vi "OAT Verify Resampled Signal (OMP, Multi Channels).vi"(0 "resampled signal":cluster{"r0":dbl, "dr":dbl, "Y":dbl[]}[](array[cluster]) {"r0" format="%.2p"; "dr" format="%.2p"; "Y" format="%.2f"}, 1 "reset in (T)":bool=TRUE, 5 "X axis selection":u16(ring)=2 items=["Time", "Revolution", "RPM"], 7 "orders to compute (1.0)":dbl[](array[numeric])=[1.0] format="%.2f", 9 "bandwidth [order]":dbl=1.0 format="%.2f", 11 "error in (no error)":errorcluster) -> (3 "reset out (T)":bool=TRUE, 4 "resampled signal out":cluster{"r0":dbl, "dr":dbl, "Y":dbl[]}[](array[cluster]), 6 "X axis selection out":u16(ring)=2 items=["Time", "Revolution", "RPM"], 8 "orders to compute (1.0) out":dbl[](array[numeric])=[1.0] format="%.2f", 10 "bandwidth [order] out":dbl=1.0 format="%.2f", 15 "error out":errorcluster)   [LabVIEW 2017, in "SoundVib_Resampling.lvlib"]
uses:
  <vilib>/addons/Sound and Vibration/Order Analysis/Resample Order Tracking/SoundVib_Resampling.lvlib
  <vilib>/addons/Sound and Vibration/Order Analysis/Resample Order Tracking/SubVIs/OAT Verify Resampled Signal (Multi Channels).vi
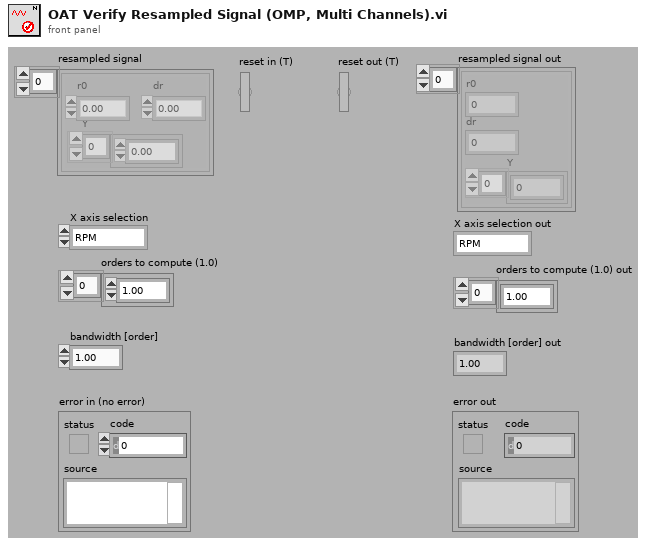
[diagram p1: front panel]
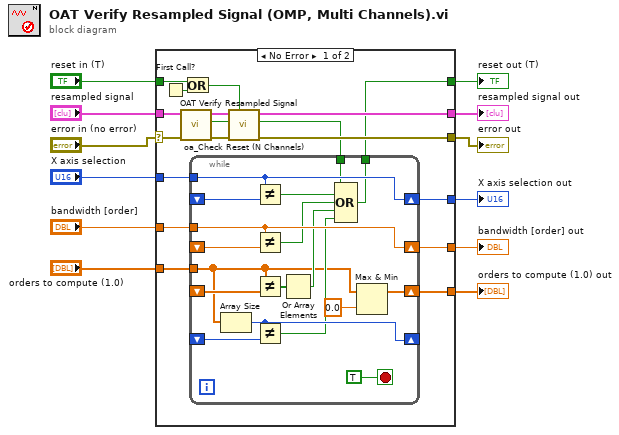
[diagram p0: block diagram]
diagram:
  n1 = case shown="No Error" "error in (no error)" {
    selector: "error in (no error)" -> [w25 w52]
    tunnel: [w23 w52] -> w12
    tunnel: [w24 w53] -> w11
    tunnel: "reset in (T)" -> [w30 w54]
    tunnel: [w13 w54] -> w9
    tunnel: "X axis selection" -> [w20 w51]
    tunnel: "orders to compute (1.0)" -> [w19 w50]
    tunnel: "bandwidth [order]" -> [w18 w49]
    tunnel: [w17 w51] -> w5
    tunnel: [w15 w50] -> w4
    tunnel: [w16 w49] -> w3
    tunnel: "resampled signal" -> [w26 w53]
    frame No Error {
      n2 = First Call?() -> (First Call?: T/F=w29:bool)
      n3 = call-poly <vilib>:"OAT Verify Resampled Signal.vi"("error in (no error)"=w25, "resampled signal"=w26) -> ("error out"=w27:errorcluster, "empty signal"=w14:bool, "resampled signal out"=w28:cluster{"r0":dbl, "dr":dbl, "Y":dbl[]}[])  [unwired: 7 in]
      n4 = Or(x=w30, y=w29) -> (x .or. y?=w22:bool)
      n5 = call <vilib>:"oa_Check Reset (N Channels).vi"("reset?"=w22, "error in (no error)"=w27, "empty?"=w14, "resampled signal"=w28) -> ("error out"=w23:errorcluster, "reset?"=w21:bool, "resampled signal out"=w24:cluster{"r0":dbl, "dr":dbl, "Y":dbl[]}[])  [unwired: 5 in]
      n6 = while {
        tunnel: w20 -> [w46]
        shift-right: [w46] -> w17
        shift-left: _ -> [w47]
        shift-right: [w44] -> w16
        shift-left: _ -> [w45]
        tunnel: w18 -> [w44]
        tunnel: w19 -> [w34]
        shift-right: [w32] -> w15
        shift-left: _ -> [w43]
        shift-right: [w40] -> _
        shift-left: _ -> [w41]
        tunnel: [w35] -> w13
        tunnel: w21 -> [w31]
        stop <- TRUE stop-if-true
        n7 = Array Size(array=w34) -> (size(s)=w40:i32)
        n8 = Not Equal?(x=w46, y=w47) -> (x != y?=w39:bool)
        n9 = Not Equal?(x=w44, y=w45) -> (x != y?=w38:bool)
        n10 = Not Equal?(x=w34, y=w43) -> (x != y?=w42:bool[])
        n11 = Not Equal?(x=w40, y=w41) -> (x != y?=w36:bool)
        n12 = Or Array Elements(Boolean array=w42) -> (logical OR=w37:bool)
        n13 = Compound Arithmetic op=OR(w31, w39, w38, w37, w36) -> (w35:bool)
        n14 = Max & Min(x=w34, y=0.0) -> (max(x,y)=w32:dbl[])  [unwired: 1 out]
      }
    }
    frame Error {
    }
  }
  "error out" <- w12
  "resampled signal out" <- w11
  "reset out (T)" <- w9
  "orders to compute (1.0) out" <- w4
  "X axis selection out" <- w5
  "bandwidth [order] out" <- w3
